vi "Launch All Modules - Top Level VI.vi"() -> ()   [LabVIEW 2018]
uses:
  modules/Common/Common.lvlib
  modules/Common/ctl/Stop All - Action.ctl
  modules/Sensor Interface/Sensor Interface.lvlib
  modules/Error Handler/Error Handler.lvlib
  modules/Controller/Controller.lvlib
  modules/User Console/User Console.lvlib
  modules/Display Console/Display Console.lvlib
panel:
  in  "error in":errorcluster
  out "error out":errorcluster
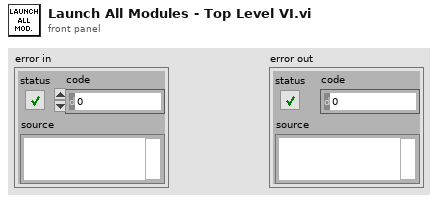
[diagram p1: front panel]
types:
  T1 = typedef "Common.lvlib/Stop All - Action.ctl" = enum16{"Create", "Fire", "Get", "Destroy"}
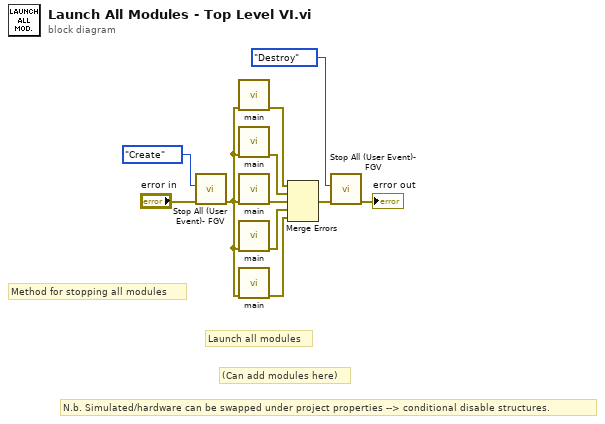
[diagram p0: block diagram]
diagram:
  # "N.b. Simulated/hardware can be swapped under project properties --> conditional disable structures."
  # "(Can add modules here)"
  # "Launch all modules"
  # "Method for stopping all modules"
  n1 = call "Stop All (User Event)- FGV.vi"("error in"="error in", "Action"=Stop_All_-_Action."Create") -> ("error out"=w9:errorcluster)  [unwired: 8 in, 1 out]
  n2 = call "main.vi"("Error in"=w9) -> ("Error out"=w8:errorcluster)  [unwired: 10 in]
  n3 = call "main.vi"("Error in"=w9) -> ("Error out"=w7:errorcluster)  [unwired: 10 in]
  n4 = call "main.vi"("Error in"=w9) -> ("Error out"=w6:errorcluster)  [unwired: 10 in]
  n5 = call "main.vi"("Error in"=w9) -> ("Error out"=w5:errorcluster)  [unwired: 10 in]
  n6 = call "main.vi"("Error in"=w9) -> ("Error out"=w4:errorcluster)  [unwired: 10 in]
  n7 = Merge Errors(w8, w7, w6, w5, w4) -> (w3:errorcluster)
  n8 = call "Stop All (User Event)- FGV.vi"("error in"=w3, "Action"=Stop_All_-_Action."Destroy") -> ("error out"=→"error out":errorcluster)  [unwired: 8 in, 1 out]
